vi "prepare buffer array seperately.vi"(7 "shots# per page":i32, 8 "error in (no error)":errorcluster, 9 "shot H":i32, 10 "page W":i32, 11 "buffer page #":i32) -> (0 "error out":errorcluster, 2 "Image array":T1[][](array[typedef]), 3 "ptr array":u64[](array[numeric]))   [LabVIEW 2021, in "Camera.lvlib" / "Camera.lvclass"]
uses:
  Camera.lvclass
  <vilib>/vision/Image Controls.llb/IMAQ Image.ctl
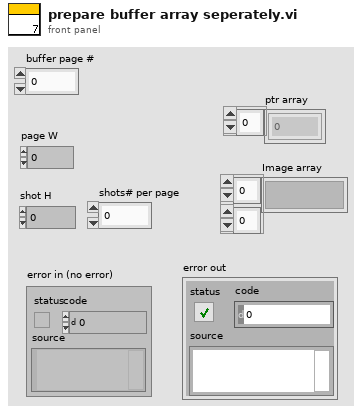
[diagram p1: front panel]
types:
  T1 = typedef "IMAQ Image.ctl" = refnum<image>
  T2 = enum32{"Map Pixel Pointer", "Unmap Pixel Pointer", "Get Pixels Infos"}
  T3 = typedef "Image Type" = u32
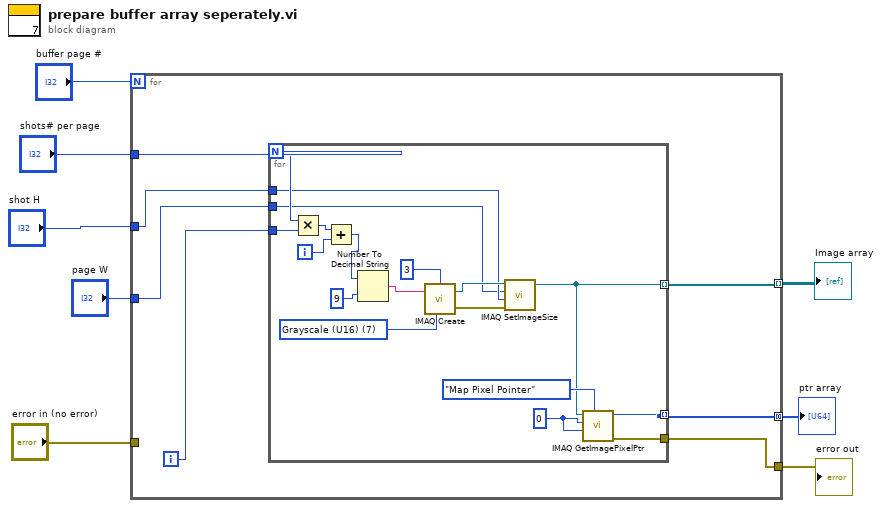
[diagram p0: block diagram]
diagram:
  n1 = for {
    N: "buffer page #" -> [_]
    tunnel: "page W" -> [w10]
    tunnel: "error in (no error)" -> [_]
    tunnel: "shots# per page" -> [w15]
    tunnel: "shot H" -> [w11]
    tunnel: [w14] -> w5 mode=concatenating
    tunnel: [w13] -> w4
    tunnel: [w9] -> w1 mode=indexing
    i -> [w12]
    n2 = for {
      N: w15 -> [w23]
      tunnel: [w32] -> w14 mode=indexing
      tunnel: [w31] -> w13
      tunnel: w12 -> [w24]
      tunnel: w11 -> [w19]
      tunnel: w10 -> [w18]
      tunnel: [w17] -> w9 mode=indexing
      i -> [w21]
      w27 = T3 7 items=["Grayscale (U8)", "Grayscale (I16)", "Grayscale (SGL)", "Complex (CSG)", "RGB (U32)", "HSL (U32)", "RGB (U64)", "Grayscale (U16)"] ("Image Type")
      w16 = 0 ("X Coordinate")
      n3 = Multiply(x=w23, y=w24) -> (x*y=w22:i32)
      n4 = Add(x=w22, y=w21) -> (x+y=w20:i32)
      n5 = Number To Decimal String(number=w20, width (-)=i16 9) -> (decimal integer string=w28:string)
      n6 = call "IMAQ Create"("Border Size"=3, "Image Name"=w28, "Image Type"=w27) -> ("New Image"=w29:T1, "error out"=w30:errorcluster)  [unwired: 2 in]
      n7 = call "IMAQ SetImageSize"("error in (no error)"=w30, "Y Resolution"=w19, "X Resolution"=w18, "Image"=w29) -> ("Image Out"=w17:T1)  [unwired: 1 in, 1 out]
      n8 = call "IMAQ GetImagePixelPtr"("Function"=T2."Map Pixel Pointer", "Y Coordinate"=w16, "X Coordinate"=w16, "Image"=w17) -> ("error out"=w31:errorcluster, "Pixel Pointer out"=w32:u64)  [unwired: 2 in, 4 out]
    }
  }
  "ptr array" <- w5
  "error out" <- w4
  "Image array" <- w1
